vi "Multiprocessing_VI_Latest.vi"() -> ()   [LabVIEW 2022 SP3]
uses:
  <vilib>/Analysis/baseanly.llb/Mean (DBL).vi
  <vilib>/DAQmx/read.llb/DAQmx Read (Analog 1D Wfm NChan NSamp).vi
  STOP_GLOBAL.vi
  <vilib>/DAQmx/configure/timing.llb/DAQmx Timing (Sample Clock).vi
  <vilib>/addons/control/pid/pid.llb/PID Gain Schedule (DBL).vi
  <vilib>/DAQmx/miscellaneous.llb/DAQmx Fill In Error Info.vi
  <resource>/objmgr/daqmx.rc
  <vilib>/addons/control/pid/NI_PID_pid.lvlib
  <vilib>/Analysis/NI_AALBase.lvlib
panel:
  in  "Manual Angle Control":dbl
  out "Voltage":dbl
  out "Waveform Graph":dbl[](graph)
  out "Voltage Command Output":dbl[](graph)
  out "VoltageSent":dbl
  out "Angle Command":dynamicdata(graph)
  in  "Ignition":bool
  in  "Stepper Voltage":ext format="%_3g"
  out "Chamber Pressure LocalVar":dynamicdata(graph)
  out "PID gains out":T1={"proportional gain (Kc)"=1.0, "integral time (Ti, min)"=0.01, "derivative time (Td, min)"=0.0} {"derivative time (Td, min)" format="%.3f"; "integral time (Ti, min)" format="%.5f"; "proportional gain (Kc)" format="%.3f"}
  out "Process Variable vs Setpoint":dynamicdata(graph)
  out "Output":dbl(slide)=30.8641975308642 scale=0.0..5.067 scale format="%.1f"
  in  "Automatic":bool=TRUE
  out "Servo/Step Voltage":dbl[](array[numeric])
  in  "SP":dbl
  in  "MV":dbl(slide)=30.8641975308642 scale=0.0..5.067 scale format="%.1f"
  in  "Stop All":bool
  out "x*y 2":dbl
  out "AI7":dynamicdata(graph)
  out "Time":dbl
  out "Inlet Thermocouple":cluster{dbl[], dbl[]}(graph)
  out "Inlet Thermocouple":dynamicdata(graph)
  out "Flow Meter Thermocouple":dynamicdata(graph)
  out "Supply P. Thermocouple":cluster{dbl[], dbl[]}(graph)
  out "Flow Meter Thermocouple":cluster{dbl[], dbl[]}(graph)
  out "Supply P. Thermocouple":dynamicdata(graph)
  out "Thrust 3":cluster{dbl[], dbl[]}(graph)
  out "Thrust 2":cluster{dbl[], dbl[]}(graph)
  out "Rocket Thrust":cluster{dbl[], dbl[]}(graph)
  out "LC3":dynamicdata(graph)
  out "LC2":dynamicdata(graph)
  out "Rocket Thrust LC1":dynamicdata(graph)
  out "Waiting \nfor Start":bool=TRUE
  in  "Start VI":bool
  out "SampClk.Rate":dbl
  in  "Sample Number":i32=100
  in  "Channel Control":bool[](array[boolean])
  in  "Rate":dbl=1000.0 format="%0.2f"
  out "AI7":cluster{dbl[], dbl[]}(graph)
  out "Vol Flow L/min":dynamicdata(graph)
  out "Process Variable vs Setpoint":cluster{dbl[], dbl[]}[](graph)
  in  "Filename":path=path "C:/1. Rocket Research Project/CollectedData/Plots/TestingData.lvm"
  in  "PID gain schedule":T2(array[cluster])=[{"PID gains"={"proportional gain (Kc)"=1.0, "integral time (Ti, min)"=0.01, "derivative time (Td, min)"=0.0}, "max value"=100.0}] {"max value" format="%.2f"; "PID gains"."derivative time (Td, min)" format="%.3f"; "PID gains"."integral time (Ti, min)" format="%.3f"; "PID gains"."proportional gain (Kc)" format="%.3f"}
  in  "Collect?":bool=TRUE caption="Enable"
  out "Vol Flow":cluster{dbl[], dbl[]}(graph)
  out "Chamber Pressure":cluster{dbl[], dbl[]}(graph)
  out "Inlet Pressure":cluster{dbl[], dbl[]}(graph)
  out "Line Pressure":cluster{dbl[], dbl[]}(graph)
  out "Supply Pressure":cluster{dbl[], dbl[]}(graph)
  out "Supply Pressure":dynamicdata(graph)
  out "Inlet Pressure":dynamicdata(graph)
  out "Line Pressure":dynamicdata(graph)
  out "Chamber Pressure PSI":dynamicdata(graph)
  out "Output Clock Rate":dbl
  out "x*y":i32
  out "error out":errorcluster
  out "Iterations":i32
  out "Angle Sensor":dynamicdata(graph)
  out "P.T. 5":dynamicdata(graph)
  # "Pressure Channels"
  # "Temperature Channels"
  # "Thrust Channels"
  # "DAQ Configuration"
  # "AI 0 - Supply Pressure"
  # "AI 1 - Flow Meter Pressure"
  # "AI 2 - Inlet Pressure"
  # "AI 3 - Chamber Pressure"
  # "AI 4 - Differential Pressure"
  # "AI 5 - Volumetric Flow"
  # "AI 6"
  # "AI 7"
  # "Load Cell 1 Right"
  # "Load Cell 2 Left"
  # "Thrust Channel 3"
  # "TC1 - Supply P. Thermocouple"
  # "TC2 - Flow Meter Thermocouple"
  # "TC3 - Inlet Thermocouple"
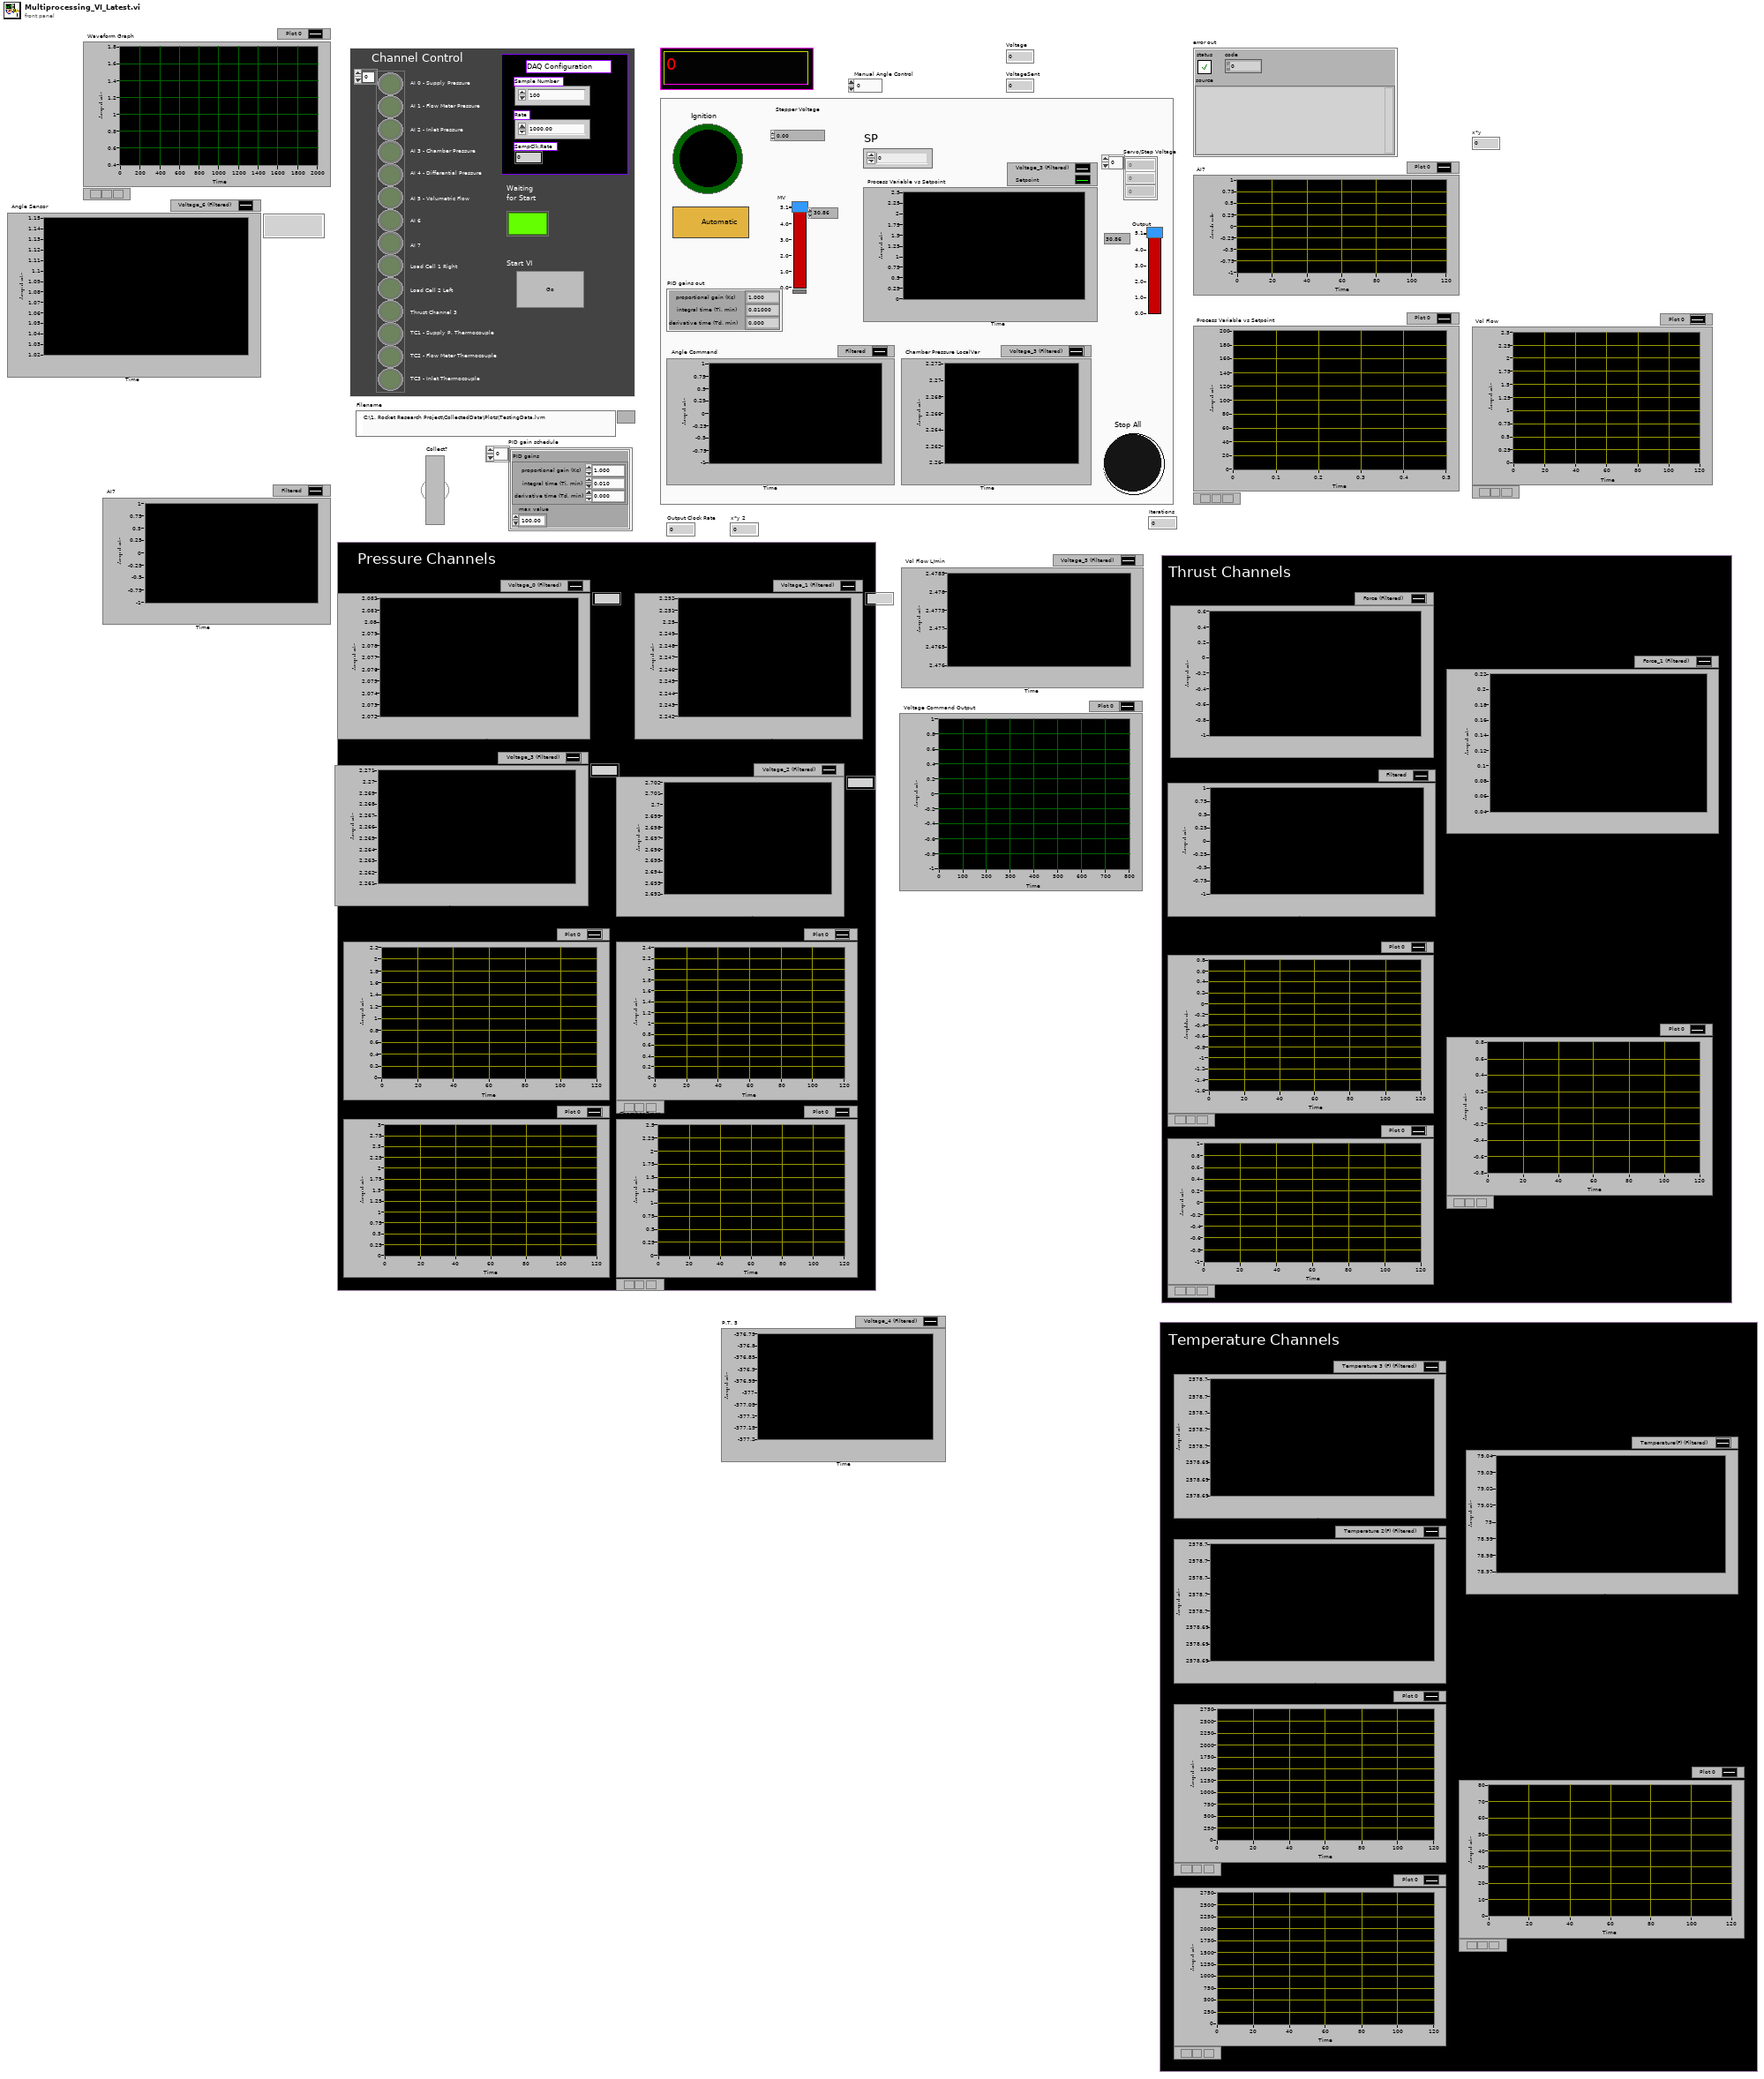
[diagram p1: front panel]
types:
  T1 = cluster{"proportional gain (Kc)":dbl, "integral time (Ti, min)":dbl, "derivative time (Td, min)":dbl}
  T2 = cluster{"PID gains":cluster{"proportional gain (Kc)":dbl, "integral time (Ti, min)":dbl, "derivative time (Td, min)":dbl}, "max value":dbl}[]
  T3 = cluster{"PID gains":cluster{"Kc":dbl, "Ti":dbl, "Td":dbl}, "max value":dbl}[]
  T4 = cluster{"Modulus":dbl, "Number of\nComplete Cycles":dbl}
  T5 = cluster{"Dynamic Data":dynamicdata, "Dynamic Data":dynamicdata, "Dynamic Data":dynamicdata, "Dynamic Data":dynamicdata, "Dynamic Data":dynamicdata, "Dynamic Data":dynamicdata, "Dynamic Data":dynamicdata, "Dynamic Data":dynamicdata, "Dynamic Data":dynamicdata, "Dynamic Data":dynamicdata, "Dynamic Data":dynamicdata, "Dynamic Data":dynamicdata, "Dynamic Data":dynamicdata, "Dynamic Data":dynamicdata}
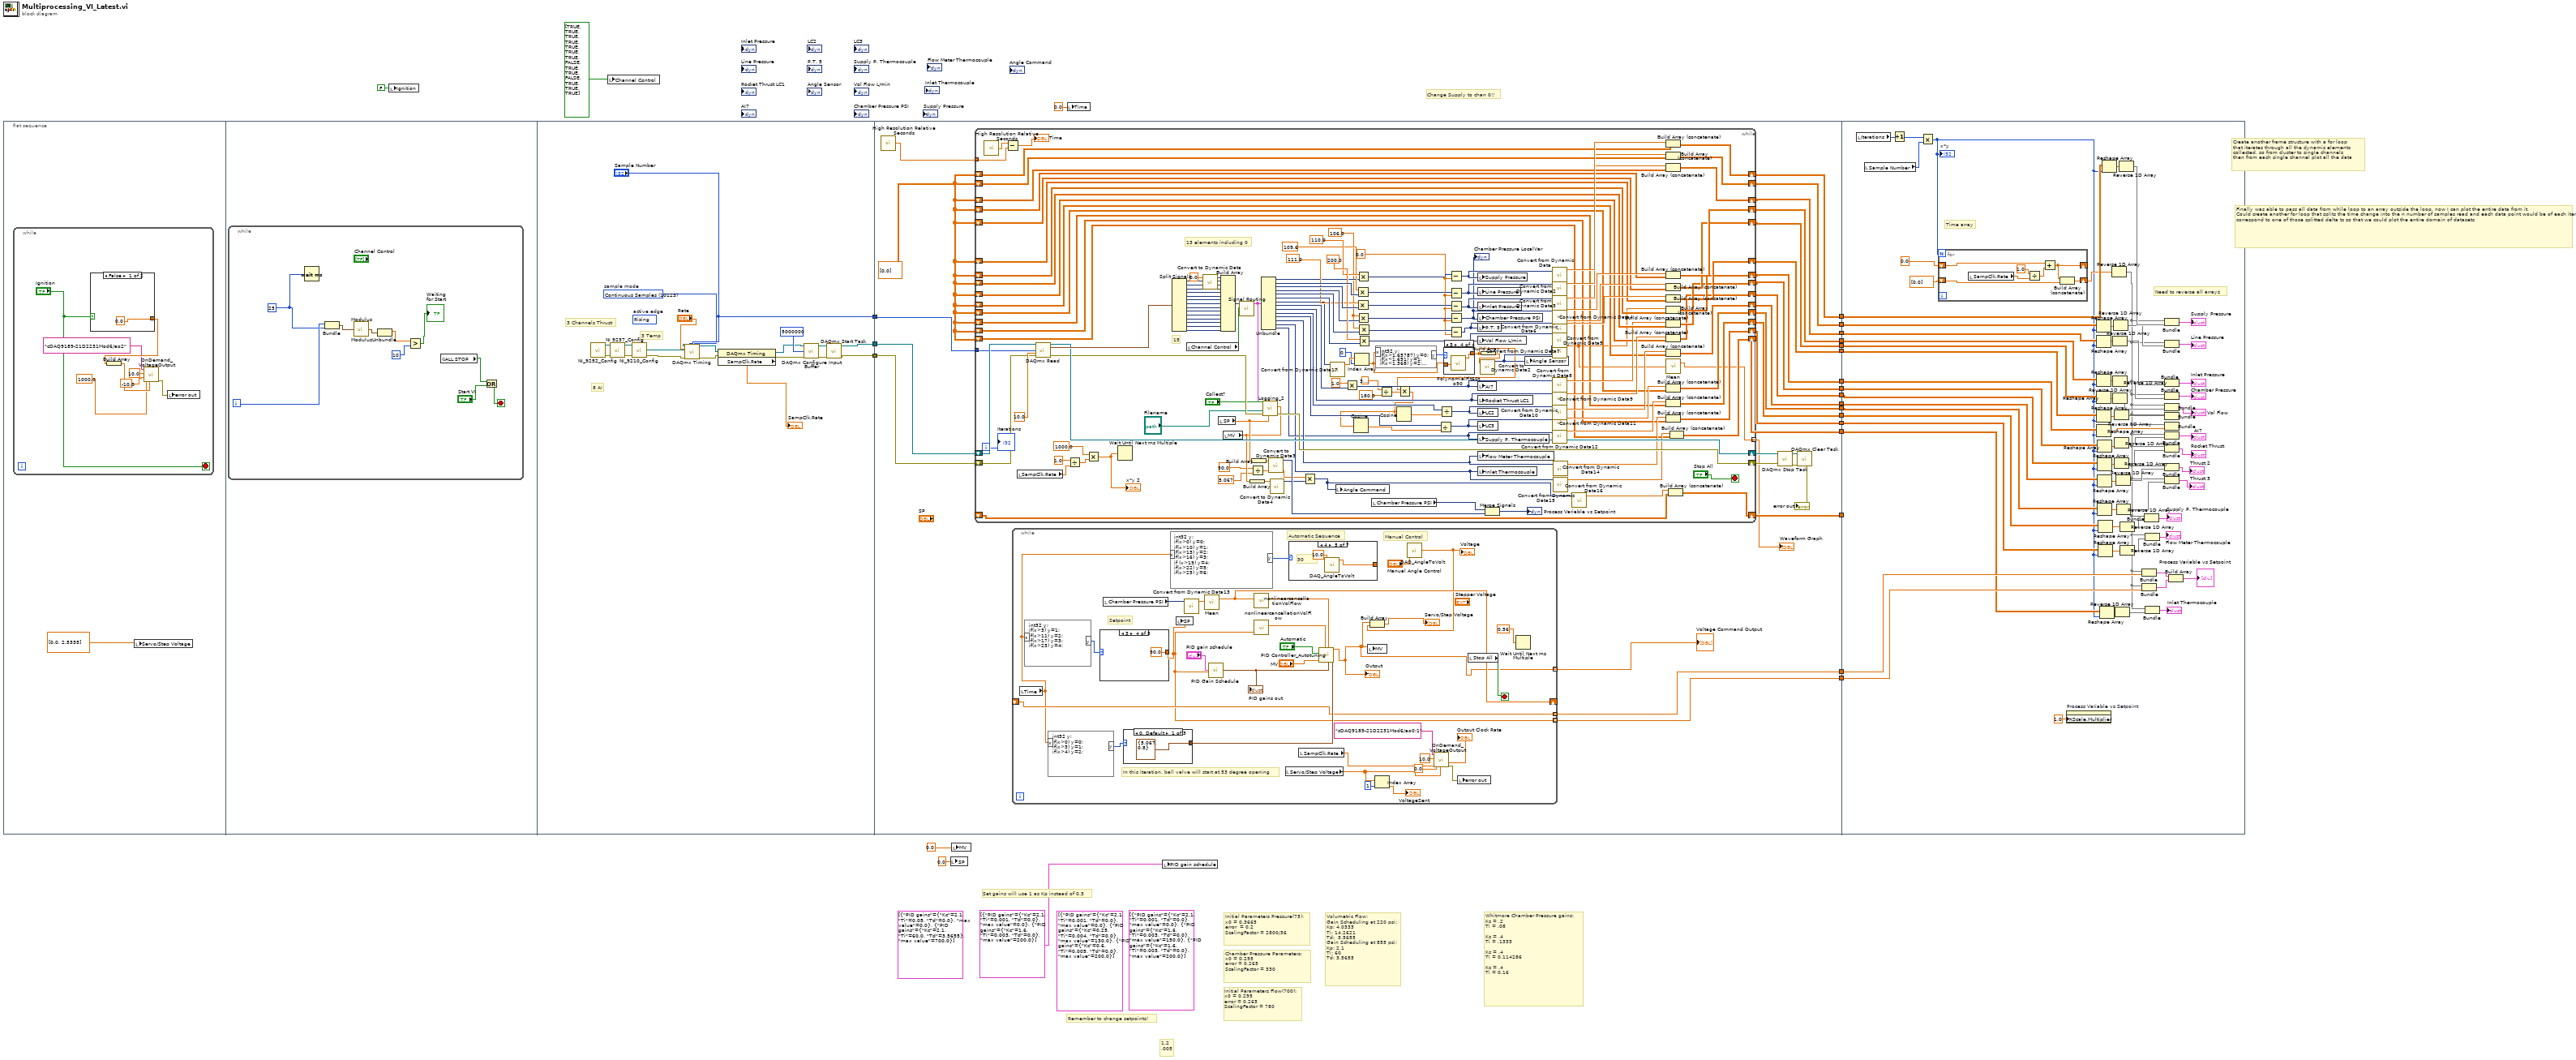
[diagram p0: block diagram]
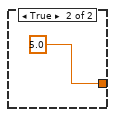
[diagram p2: hidden frame]
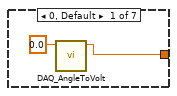
[diagram p3: hidden frame]
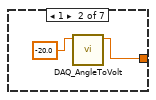
[diagram p4: hidden frame]
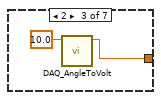
[diagram p5: hidden frame]
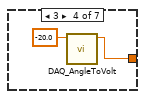
[diagram p6: hidden frame]
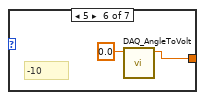
[diagram p7: hidden frame]
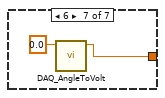
[diagram p8: hidden frame]
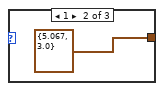
[diagram p9: hidden frame]
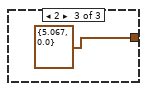
[diagram p10: hidden frame]
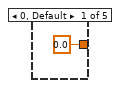
[diagram p11: hidden frame]
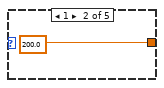
[diagram p12: hidden frame]
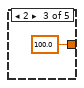
[diagram p13: hidden frame]
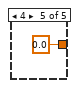
[diagram p14: hidden frame]
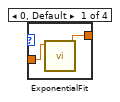
[diagram p15: hidden frame]
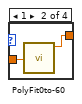
[diagram p16: hidden frame]
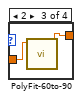
[diagram p17: hidden frame]
diagram:
  (unwired) T3 [{"PID gains"={"Kc"=2.1, "Ti"=0.001, "Td"=0.0}, "max value"=0.0}, {"PID gains"={"Kc"=1.6, "Ti"=0.003, "Td"=0.0}, "max value"=150.0}, {"PID gains"={"Kc"=1.6, "Ti"=0.003, "Td"=0.0}, "max value"=200.0}]
  (unwired) T3 [{"PID gains"={"Kc"=2.1, "Ti"=0.001, "Td"=0.0}, "max value"=0.0}, {"PID gains"={"Kc"=0.25, "Ti"=0.004, "Td"=0.0}, "max value"=130.0}, {"PID gains"={"Kc"=0.6, "Ti"=0.005, "Td"=0.0}, "max value"=200.0}]
  (unwired) T3 [{"PID gains"={"Kc"=2.1, "Ti"=0.05, "Td"=0.0}, "max value"=0.0}, {"PID gains"={"Kc"=2.1, "Ti"=60.0, "Td"=3.5655}, "max value"=700.0}]
  # "1.2\n.005"
  # "Set gains will use 1 as Kp instead of 0.3"
  # "Remember to change setpoints!"
  # "Whitmore Chamber Pressure gains:\nKc = .2\nTi = .08\n\nKc = .4\nTi = .1333\n\nKc = .4\nTi = 0.114286\n\nKc = .4\nTi = 0.16"
  # "Chamber Pressure Parameters:\nx0 = 0.295\nerror = 0.265\nScalingFactor = 330"
  # "Volumetric Flow:\nGain Scheduling at 220 psi:\nKp: 4.0333\nTi: 14.2621\nTd:  3.5655\nGain Scheduling at 855 psi:\nKp: 2.1\nTi: 60\nTd: 3.5655"
  # "Initial Parameters Flow(700):\nx0 = 0.295\nerror = 0.265\nScalingFactor = 780"
  # "Initial Parameters Pressure(75):\nx0 = 0.3665\nerror  = 0.2\nScalingFactor = 2800/36"
  # "Change Supply to chan 0!!"
  # "Finally was able to pass all data from while loop to an array outside the loop, now I can plot the entire data from it, \nCould create another for loop that splits the time change into the n number of samples read and each data point would be of each iteration would correspond to one of those splitted delta ts so that we could plot the entire domain of datasets"
  # "Create another frame structure with a for loop\nthat iterates through all the dynamic elements\ncollected, so from cluster to single channels\nthen from each single channel plot all the data"
  n1 = flat-sequence {
    tunnel: [w59] -> w25
    tunnel: [w48] -> w24
    tunnel: ["Sample Number"] -> w4
    tunnel: w25 -> [w95]
    tunnel: w24 -> [w94]
    tunnel: [w87] -> w23
    tunnel: [w86] -> w21
    tunnel: [w85] -> w20
    tunnel: [w84] -> w19
    tunnel: [w83] -> w18
    tunnel: [w82] -> w17
    tunnel: [w81] -> w16
    tunnel: [w80] -> w15
    tunnel: [w79] -> w14
    tunnel: [w78] -> w13
    tunnel: [w77] -> w12
    tunnel: [w76] -> w11
    tunnel: [w75] -> w9
    tunnel: [w74] -> w8
    tunnel: [w72] -> w6
    tunnel: [w71] -> w5
    tunnel: w4 -> [w70]
    tunnel: [w69] -> w2
    tunnel: w23 -> [w363]
    tunnel: w21 -> [w362]
    tunnel: w20 -> [w361]
    tunnel: w19 -> [w360]
    tunnel: w18 -> [w359]
    tunnel: w17 -> [w358]
    tunnel: w16 -> [w357]
    tunnel: w15 -> [w355]
    tunnel: w14 -> [w354]
    tunnel: w13 -> [w353]
    tunnel: w12 -> [w352]
    tunnel: w11 -> [w351]
    tunnel: w9 -> [w346]
    tunnel: w8 -> [w345]
    tunnel: w6 -> [w320]
    tunnel: w5 -> [w319]
    tunnel: w2 -> [_]
    frame #0 {
      n2 = while {
        stop <- "Ignition" stop-if-true
        n3 = case shown="False" "Ignition" {
          tunnel: [0.0 ("element") 5.0 ("element")] -> w34
          frame False {
          }
          frame True {
          }
        }
        n4 = Build Array(w34) -> (w35:dbl[])
        n5 = call "OnDemand_VoltageOutput.vi"("Channel Array"=w35, "SampClk.Rate 2"=1000.0, "minimum voltage"=-10.0, "maximum voltage"=10.0, "physical channels"="cDAQ9189-21D2231Mod6/ao2") -> ("error out"=w33:errorcluster)  [unwired: 4 in, 2 out]
        n6 = local write "error out"(w33) -> ()
      }
      n7 = local write "Servo/Step Voltage"(dbl[] [0.0, 2.5335] ("Servo/Step Voltage")) -> ()
    }
    frame #1 {
      n8 = while {
        i -> [w47]
        stop <- w39 stop-if-true
        w38 = u32 25 ("milliseconds to wait")
        n9 = Wait (ms)(milliseconds to wait=w38) -> ()  [unwired: 1 out]
        n10 = Bundle(w47, "milliseconds to wait"=w38) -> (w46:cluster{i32, "milliseconds to wait":u32})  [unwired: 1 in]
        n11 = call "Modulus.vi"("Input"=w46) -> ("Output"=w45:T4)
        n12 = call "Modulus.vi"() -> ()  [unwired: 1 in, 1 out]
        n13 = Unbundle(w45) -> ("Modulus"=w44:dbl)  [unwired: 1 out]
        n14 = Greater?(x=w44, y=u32 10 ("milliseconds to wait")) -> (0:→"Waiting \nfor Start":bool)
        n15 = global read "STOP_GLOBAL.vi" "ALL STOP"() -> (w41:bool)
        n16 = Or(x=w41, y="Start VI") -> (x .or. y?=w39:bool)
      }
    }
    frame #2 {
      w50 = 10123 items=["Finite Samples"=10178, "Continuous Samples"=10123, "Hardware Timed Single Point"=12522]  # sample mode
      (unwired) 10280 items=["Rising"=10280, "Falling"=10171]  # active edge
      # "3 Temp"
      # "8 AI"
      # "3 Channels Thrust"
      n17 = call "NI_9252_Config.vi"() -> ("error out"=w57:errorcluster, "task out"=w58:refnum<k21>)  [unwired: 10 in]
      n18 = call "NI 9237_Config.vi"("error in"=w57, "task in"=w58) -> ("error out"=w66:errorcluster, "task out"=w65:refnum<k21>)  [unwired: 8 in]
      n19 = call "NI_9210_Config.vi"("error in"=w66, "task in"=w65) -> ("error out"=w53:errorcluster, "task out"=w55:refnum<k21>)  [unwired: 8 in]
      n20 = call-poly <vilib>:"DAQmx Timing.vi"("task/channels in"=w55, "sample mode"=w50, "samples per channel"="Sample Number", "rate"="Rate", "error in"=w53) -> ("task out"=w51:refnum<k21>, "error out"=w52:errorcluster)  [unwired: 9 in]
      n21 = property class="DAQmx Timing"(reference=w51, error in=w52) -> (reference out=w49:refnum<k21>, error out=w62:errorcluster, "SampClk.Rate"=→"SampClk.Rate":dbl)
      n22 = call <vilib>:"DAQmx Configure Input Buffer.vi"("task/channels in"=w49, "buffer size (in samples per channel)"=u32 5000000, "error in"=w62) -> ("task out"=w64:refnum<k21>, "error out"=w63:errorcluster)  [unwired: 11 in]
      n23 = call <vilib>:"DAQmx Start Task.vi"("task/channels in"=w64, "error in"=w63) -> ("task out"=w59:refnum<k21>, "error out"=w48:errorcluster)  [unwired: 12 in]
    }
    frame #3 {
      w73 = dbl[][] [[0.0]]
      n24 = call <vilib>:"High Resolution Relative Seconds.vi"() -> ("relative seconds"=w93:dbl)
      n25 = while {
        shift-right: [w289] -> w89
        shift-left: w95 -> [w291]
        shift-right: [w267] -> w88
        shift-left: w94 -> [w290]
        shift-right: [w178] -> w87
        shift-left: w73 -> [w227]
        tunnel: w93 -> [w264]
        shift-right: [w258] -> w86
        shift-left: w73 -> [w259]
        shift-right: [w254] -> w85
        shift-left: w73 -> [w255]
        shift-right: [w252] -> w84
        shift-left: w73 -> [w253]
        shift-right: [w250] -> w83
        shift-left: w73 -> [w249]
        shift-right: [w247] -> w82
        shift-left: w73 -> [w245]
        shift-right: [w246] -> w81
        shift-left: w73 -> [w244]
        shift-right: [w243] -> w80
        shift-left: w73 -> [w242]
        shift-right: [w237] -> w79
        shift-left: w73 -> [w236]
        shift-right: [w235] -> w78
        shift-left: w73 -> [w234]
        shift-right: [w232] -> w77
        shift-left: w73 -> [w231]
        shift-right: [w229] -> w76
        shift-left: w73 -> [w228]
        shift-right: [w206] -> w72
        shift-left: w73 -> [w205]
        shift-right: [w202] -> w71
        shift-left: w73 -> [w203]
        tunnel: w70 -> [w199]
        shift-right: [w173] -> w69
        shift-left: _ -> [w174]
        tunnel: [w167] -> w67 mode=indexing
        i -> [w266]
        stop <- "Stop All" stop-if-true
        w169 = 106.0 ("x")
        w191 = 0.0 ("y")
        # "13 elements including 0"
        # "15"
        n26 = call <vilib>:"High Resolution Relative Seconds.vi"() -> ("relative seconds"=w265:dbl)
        n27 = Subtract(x=w265, y=w264) -> (x-y=→"Time":dbl)
        n28 = local read "SampClk.Rate"() -> (w224:dbl)
        n29 = call-poly <vilib>:"DAQmx Read.vi"("task/channels in"=w291, "number of samples per channel"=w199, "timeout"=10.0, "error in"=w290) -> ("task out"=w289:refnum<k21>, "data"=w292:waveform(dbl)[], "error out"=w269:errorcluster)  [unwired: 9 in]
        n30 = Divide(x=1.0, y=w224) -> (x/y=w223:dbl)
        n31 = Multiply(x=1000.0, y=w223) -> (x*y=w221:dbl)
        "x*y 2" <- w221
        n32 = Wait Until Next ms Multiple(millisecond multiple=w221) -> ()  [unwired: 1 out]
        n33 = Split Signals(w292) -> (w283:dynamicdata, w288:dynamicdata, w287:dynamicdata, w286:dynamicdata, w285:dynamicdata, w284:dynamicdata, w282:dynamicdata, w281:dynamicdata, w280:dynamicdata, w279:dynamicdata, w278:dynamicdata, w275:dynamicdata, w209:dynamicdata, w208:dynamicdata)  [unwired: 14 in]
        n34 = local read "Channel Control"() -> (w274:bool[])
        n35 = call "Convert to Dynamic Data"("Double"=0.0) -> ("Dynamic Data Type"=w276:dynamicdata)  [unwired: 3 in]
        n36 = local read "SP"() -> (w189:dbl)
        n37 = Build Array(w276, w283, w288, w287, w286, w285, w284, w282, w281, w280, w279, w278, w275, w209, w208) -> (w273:dynamicdata[])
        n38 = local read "MV"() -> (w184:dbl)
        n39 = call "Signal Routing.vi"("Boolean Array"=w274, "Data In"=w273) -> ("Output"=w198:T5)  [unwired: 9 in]
        n40 = Build Array(w184) -> (w183:dbl[])
        n41 = Divide(x=90.0, y=5.067) -> (x/y=w172:dbl)
        n42 = Build Array(w189) -> (w188:dbl[])
        n43 = Unbundle(w198) -> ("Dynamic Data"=w177:dynamicdata, "Dynamic Data"=w272:dynamicdata, "Dynamic Data"=w271:dynamicdata, "Dynamic Data"=w190:dynamicdata, "Dynamic Data"=w270:dynamicdata, "Dynamic Data"=w201:dynamicdata, "Dynamic Data"=w155:dynamicdata, "Dynamic Data"=w220:dynamicdata, "Dynamic Data"=w241:dynamicdata, "Dynamic Data"=w160:dynamicdata, "Dynamic Data"=w157:dynamicdata, "Dynamic Data"=w197:dynamicdata, "Dynamic Data"=w195:dynamicdata, "Dynamic Data"=w196:dynamicdata)
        n44 = call "Logging_2.vi"("Voltage Command"=w184, "Setpoint"=w189, "error in"=w269, "Filename"="Filename", "Enable"="Collect?", "output cluster"=w198) -> ("error out"=w267:errorcluster)  [unwired: 5 in]
        n45 = call "Convert to Dynamic Data3"("Array"=w188) -> ("Dynamic Data Type"=w187:dynamicdata)  [unwired: 3 in]
        n46 = call "Convert to Dynamic Data4"("Array"=w183) -> ("Dynamic Data Type"=w182:dynamicdata)  [unwired: 3 in]
        n47 = Multiply(x=w172, y=w182) -> (x*y=w176:dynamicdata)
        n48 = call "Convert from Dynamic Data17"("Dynamic Data Type"=w155) -> ("Array"=w165:dbl[])  [unwired: 3 in]
        n49 = local write "Angle Command"(w176) -> ()
        n50 = Multiply(x=1.0, y=w220) -> (x*y=w218:dynamicdata)
        n51 = Index Array(array=w165, index=0) -> (element=w162:dbl)
        n52 = Multiply(x=109.6, y=w272) -> (x*y=w216:dynamicdata)
        n53 = Multiply(x=111.0, y=w271) -> (x*y=w217:dynamicdata)
        n54 = Multiply(x=110.0, y=w177) -> (x*y=w215:dynamicdata)
        n55 = Multiply(x=w169, y=w190) -> (x*y=w211:dynamicdata)
        n56 = Multiply(x=w169, y=w270) -> (x*y=w193:dynamicdata)
        n57 = Multiply(x=200.0, y=w201) -> (x*y=w194:dynamicdata)
        n58 = local read "Chamber Pressure PSI"() -> (w185:dynamicdata)
        n59 = formula code="int32 y;\nif(x>1.65787) y=0;\nif(x<1.651) y=1;\nif(x<1.368) y=2;\nif(x>1.935) y=3;"("x"=w162) -> ("y"=w166:i32)
        n60 = Divide(x=3.141592653589793, y=180.0 ("x")) -> (x/y=w151:dbl)
        n61 = case shown="3" w166 {
          tunnel: w162 -> [w295 w297 w299 w301]
          tunnel: [w294 w296 w298 w300] -> w150
          frame 0, Default {
            n62 = call "ExponentialFit.vi"("voltage"=w295) -> ("angle"=w294:dbl)  [unwired: 10 in]
          }
          frame 1 {
            n63 = call "PolyFit0to-60.vi"("input variable"=w297) -> ("output variable"=w296:dbl)  [unwired: 10 in]
          }
          frame 2 {
            n64 = call "PolyFit-60to-90.vi"("Voltage"=w299) -> ("Angle"=w298:dbl)  [unwired: 10 in]
          }
          frame 3 {
            n65 = call "PolynomialFit60to90.vi"("voltage"=w301) -> ("Angle"=w300:dbl)  [unwired: 10 in]
          }
        }
        n66 = Multiply(x=w150, y=w151) -> (x*y=w149:dbl)
        n67 = Cosine(x=w149) -> (cos(x)=w158:dbl)
        n68 = Cosine(x=w149) -> (cos(x)=w161:dbl)
        n69 = Divide(x=w157, y=w158) -> (x/y=w156:dynamicdata)
        n70 = Divide(x=w160, y=w161) -> (x/y=w159:dynamicdata)
        n71 = Subtract(x=w215, y=w191) -> (x-y=w214:dynamicdata)
        n72 = Subtract(x=w216, y=w191) -> (x-y=w213:dynamicdata)
        n73 = Subtract(x=w217, y=w191) -> (x-y=w212:dynamicdata)
        n74 = Subtract(x=w211, y=w191) -> (x-y=w210:dynamicdata)
        "Chamber Pressure LocalVar" <- w210
        n75 = Subtract(x=w193, y=w191) -> (x-y=w192:dynamicdata)
        n76 = local write "Supply Pressure"(w214) -> ()
        n77 = local write "Line Pressure"(w213) -> ()
        n78 = local write "Inlet Pressure"(w212) -> ()
        n79 = local write "Chamber Pressure PSI"(w210) -> ()
        n80 = local write "P.T. 5"(w192) -> ()
        n81 = local write "Vol Flow L/min"(w194) -> ()
        n82 = local write "AI7"(w218) -> ()
        n83 = local write "Rocket Thrust LC1"(w241) -> ()
        n84 = local write "LC2"(w159) -> ()
        n85 = local write "LC3"(w156) -> ()
        n86 = local write "Supply P. Thermocouple"(w196) -> ()
        n87 = local write "Flow Meter Thermocouple"(w197) -> ()
        n88 = local write "Inlet Thermocouple"(w195) -> ()
        n89 = Build Array(w150) -> (w163:dbl[])
        n90 = call "Convert to Dynamic Data2"("Array"=w163) -> ("Dynamic Data Type"=w154:dynamicdata)  [unwired: 3 in]
        n91 = Merge Signals(w185, w187) -> (→"Process Variable vs Setpoint":dynamicdata)
        n92 = local write "Angle Sensor"(w154) -> ()
        n93 = call "Convert from Dynamic Data"("Dynamic Data Type"=w214) -> ("Array"=w263:dbl[])  [unwired: 3 in]
        n94 = call "Convert from Dynamic Data2"("Dynamic Data Type"=w213) -> ("Array"=w260:dbl[])  [unwired: 3 in]
        n95 = call "Convert from Dynamic Data3"("Dynamic Data Type"=w212) -> ("Array"=w257:dbl[])  [unwired: 3 in]
        n96 = call "Convert from Dynamic Data4"("Dynamic Data Type"=w210) -> ("Array"=w256:dbl[])  [unwired: 3 in]
        n97 = call "Convert from Dynamic Data6"("Dynamic Data Type"=w192) -> ("Array"=w248:dbl[])  [unwired: 3 in]
        n98 = call "Convert from Dynamic Data5"("Dynamic Data Type"=w194) -> ("Array"=w251:dbl[])  [unwired: 3 in]
        n99 = call "Convert from Dynamic Data7"("Dynamic Data Type"=w154) -> ("Array"=w168:dbl[])  [unwired: 3 in]
        n100 = call "Convert from Dynamic Data8"("Dynamic Data Type"=w218) -> ("Array"=w240:dbl[])  [unwired: 3 in]
        n101 = call "Convert from Dynamic Data9"("Dynamic Data Type"=w241) -> ("Array"=w239:dbl[])  [unwired: 3 in]
        n102 = call "Convert from Dynamic Data10"("Dynamic Data Type"=w159) -> ("Array"=w238:dbl[])  [unwired: 3 in]
        n103 = call "Convert from Dynamic Data11"("Dynamic Data Type"=w156) -> ("Array"=w233:dbl[])  [unwired: 3 in]
        n104 = call "Convert from Dynamic Data12"("Dynamic Data Type"=w196) -> ("Array"=w230:dbl[])  [unwired: 3 in]
        n105 = call "Convert from Dynamic Data14"("Dynamic Data Type"=w197) -> ("Array"=w207:dbl[])  [unwired: 3 in]
        n106 = call "Convert from Dynamic Data15"("Dynamic Data Type"=w195) -> ("Array"=w204:dbl[])  [unwired: 3 in]
        n107 = call "Convert from Dynamic Data16"("Dynamic Data Type"=w176) -> ("Array"=w175:dbl[])  [unwired: 3 in]
        n108 = Build Array (concatenate)(w263, w227) -> (w178:dbl[][])
        n109 = Build Array (concatenate)(w260, w259) -> (w258:dbl[][])
        n110 = Build Array (concatenate)(w257, w255) -> (w254:dbl[][])
        n111 = Build Array (concatenate)(w256, w253) -> (w252:dbl[][])
        n112 = Build Array (concatenate)(w251, w249) -> (w250:dbl[][])
        n113 = Build Array (concatenate)(w248, w245) -> (w247:dbl[][])
        n114 = Build Array (concatenate)(w168, w244) -> (w246:dbl[][])
        n115 = Build Array (concatenate)(w240, w242) -> (w243:dbl[][])
        n116 = Build Array (concatenate)(w239, w236) -> (w237:dbl[][])
        n117 = Build Array (concatenate)(w238, w234) -> (w235:dbl[][])
        n118 = Build Array (concatenate)(w233, w231) -> (w232:dbl[][])
        n119 = Build Array (concatenate)(w230, w228) -> (w229:dbl[][])
        n120 = call-poly <vilib>:"Mean.vi"("X"=w168) -> ("mean"=w167:dbl)  [unwired: 1 out]
        n121 = Build Array (concatenate)(w207, w205) -> (w206:dbl[][])
        n122 = Build Array (concatenate)(w175, w174) -> (w173:dbl[][])
        n123 = Build Array (concatenate)(w204, w203) -> (w202:dbl[][])
        "Iterations" <- w266
      }
      "Waveform Graph" <- w67
      n124 = while {
        shift-right: [w118] -> _
        shift-left: _ -> [w114]
        tunnel: [w114] -> w75 mode=indexing
        tunnel: [w106] -> w74 mode=indexing
        tunnel: [w98] -> w68 mode=indexing
        stop <- w121 stop-if-true
        # "Manual Control"
        # "Automatic Sequence"
        # "In this iteration, ball valve will start at 53 degree opening"
        # "Setpoint"
        n125 = local read "Time"() -> (w103:dbl)
        n126 = formula code="int32 y;\nif(x>3) y=1;\nif(x>11) y=2;\nif(x>17) y=3;\nif(x>23) y=4;"("x"=w103) -> ("y"=w117:i32)
        n127 = formula code="int32 y;\nif(x>0) y=0;\nif(x>3) y=1;\nif(x>4) y=2;"("x"=w103) -> ("y"=w116:i32)
        n128 = case shown="3" w117 {
          tunnel: [0.0 ("SP") 200.0 ("SP") 100.0 ("SP") 90.0 ("SP") 0.0 ("SP")] -> w106
          frame 0, Default {
          }
          frame 1 {
          }
          frame 2 {
          }
          frame 3 {
          }
          frame 4 {
          }
        }
        n129 = local read "Chamber Pressure PSI"() -> (w105:dynamicdata)
        n130 = case shown="0, Default" w116 {
          tunnel: [cluster{"output high":dbl, "output low":dbl} {"output high"=5.067, "output low"=0.8} ("output range") cluster{"output high":dbl, "output low":dbl} {"output high"=5.067, "output low"=3.0} ("output range") cluster{"output high":dbl, "output low":dbl} {"output high"=5.067, "output low"=0.0} ("output range")] -> w115
          frame 0, Default {
          }
          frame 1 {
          }
          frame 2 {
          }
        }
        n131 = formula code="int32 y;\nif(x>0) y=0;\nif(x>10) y=1;\nif(x>13) y=2;\nif(x>16) y=3;\nif (x>19) y=4;\nif(x>22) y=5;\nif(x>25) y=6;"("x"=w103) -> ("y"=w102:i32)
        n132 = local write "SP"(w106) -> ()
        n133 = call "Convert from Dynamic Data13"("Dynamic Data Type"=w105) -> ("Array"=w119:dbl[])  [unwired: 3 in]
        n134 = call-poly <vilib>:"Mean.vi"("X"=w119) -> ("mean"=w118:dbl)  [unwired: 1 out]
        n135 = call-poly <vilib>:"PID Gain Schedule.vi"("PID gain schedule"="PID gain schedule", "gain scheduling value"=w106) -> ("PID gains out"=w125:T1)  [unwired: 2 in, 1 out]
        "PID gains out" <- w125
        n136 = call "nonlinearcancellationVolFlow.vi"("input variable"=w118) -> ("MVT Process Variable"=w120:dbl)  [unwired: 10 in]
        n137 = call "nonlinearcancellationVolFlow.vi"("input variable"=w106) -> ("MVT Process Variable"=w123:dbl)  [unwired: 10 in]
        n138 = local read "Servo/Step Voltage"() -> (w101:dbl[])
        n139 = case shown="4" w102 {
          tunnel: [w128 w129 w131 w134 w135 w138 w139] -> _
          frame 0, Default {
            n140 = call "DAQ_AngleToVolt.vi"("Angle"=0.0) -> ("Voltage"=w128:dbl)  [unwired: 10 in]
          }
          frame 1 {
            n141 = call "DAQ_AngleToVolt.vi"("Angle"=-20.0 ("x")) -> ("Voltage"=w129:dbl)  [unwired: 10 in]
          }
          frame 2 {
            n142 = call "DAQ_AngleToVolt.vi"("Angle"=10.0) -> ("Voltage"=w131:dbl)  [unwired: 10 in]
          }
          frame 3 {
            n143 = call "DAQ_AngleToVolt.vi"("Angle"=-20.0) -> ("Voltage"=w134:dbl)  [unwired: 10 in]
          }
          frame 4 {
            # "30"
            n144 = call "DAQ_AngleToVolt.vi"("Angle"=10.0) -> ("Voltage"=w135:dbl)  [unwired: 10 in]
          }
          frame 5 {
            # "-10"
            n145 = call "DAQ_AngleToVolt.vi"("Angle"=0.0) -> ("Voltage"=w138:dbl)  [unwired: 10 in]
          }
          frame 6 {
            n146 = call "DAQ_AngleToVolt.vi"("Angle"=0.0) -> ("Voltage"=w139:dbl)  [unwired: 10 in]
          }
        }
        n147 = local read "SampClk.Rate"() -> (w112:dbl)
        n148 = call "PID Controller_Autotuning.vi"("output range"=w115, "PID gains in"=w125, "process variable"=w120, "setpoint"=w123, "manipulated variable"="MV", "Automatic"="Automatic") -> ("output"=w98:dbl)  [unwired: 4 in, 1 out]
        "Output" <- w98
        n149 = local write "MV"(w98) -> ()
        n150 = Index Array(array=w101, index=1) -> (element=→"VoltageSent":dbl)
        n151 = call "DAQ_AngleToVolt.vi"("Angle"="Manual Angle Control") -> ("Voltage"=w96:dbl)  [unwired: 10 in]
        "Voltage" <- w96
        n152 = Build Array(w98, w96) -> (→"Servo/Step Voltage":dbl[])
        n153 = call "OnDemand_VoltageOutput.vi"("Channel Array"=w101, "SampClk.Rate 2"=w112, "minimum voltage"=0.0, "maximum voltage"=10.0, "physical channels"="cDAQ9189-21D2231Mod6/ao0:1") -> ("error out"=w111:errorcluster, "SampClk.Rate"=→"Output Clock Rate":dbl)  [unwired: 4 in, 1 out]
        n154 = local write "error out"(w111) -> ()
        n155 = local read "Stop All"() -> (w121:bool)
        n156 = Wait Until Next ms Multiple(millisecond multiple=0.56 ("x")) -> ()  [unwired: 1 out]
      }
      "Voltage Command Output" <- w68
      n157 = call <vilib>:"DAQmx Stop Task.vi"("task/channels in"=w89, "error in"=w88) -> ("task out"=w92:refnum<k21>, "error out"=w91:errorcluster)  [unwired: 12 in]
      n158 = call <vilib>:"DAQmx Clear Task.vi"("task in"=w92, "error in"=w91) -> ("error out"=→"error out":errorcluster)  [unwired: 13 in]
    }
    frame #4 {
      # "Time array"
      # "Need to reverse all arrays"
      n159 = local read "Iterations"() -> (w368:i32)
      n160 = local read "Sample Number"() -> (w304:i32)
      n161 = Increment(x=w368) -> (x+1=w367:i32)
      n162 = Multiply(x=w367, y=w304) -> (x*y=w303:i32)
      "x*y" <- w303
      n163 = for {
        N: w303 -> [_]
        shift-right: [w371] -> _
        shift-left: 0.0 -> [w372]
        shift-right: [w370] -> w341
        shift-left: dbl[] [0.0] -> [w369]
        n164 = local read "SampClk.Rate"() -> (w374:dbl)
        n165 = Divide(x=1.0, y=w374) -> (x/y=w373:dbl)
        n166 = Add(x=w372, y=w373) -> (x+y=w371:dbl)
        n167 = Build Array (concatenate)(w371, w369) -> (w370:dbl[])
      }
      n168 = property on="Process Variable vs Setpoint" class="XYGraph (strict)"("XScale.Multiplier"=1.0 ("X Scale.Offset and Multiplier:Multiplier")) -> ()  [unwired: 2 in, 2 out]
      n169 = Reshape Array(w362, w303) -> (w337:dbl[])
      n170 = Reshape Array(w361, w303) -> (w335:dbl[])
      n171 = Reshape Array(w360, w303) -> (w333:dbl[])
      n172 = Reshape Array(w359, w303) -> (w331:dbl[])
      n173 = Reshape Array(w358, w303) -> (w329:dbl[])
      n174 = Reshape Array(w357, w303) -> (w356:dbl[])
      n175 = Reshape Array(w355, w303) -> (w326:dbl[])
      n176 = Reshape Array(w353, w303) -> (w310:dbl[])
      n177 = Reshape Array(w354, w303) -> (w318:dbl[])
      n178 = Reshape Array(w352, w303) -> (w307:dbl[])
      n179 = Reshape Array(w351, w303) -> (w323:dbl[])
      n180 = Reshape Array(w320, w303) -> (w316:dbl[])
      n181 = Reshape Array(w319, w303) -> (w311:dbl[])
      n182 = Reshape Array(w363, w303) -> (w339:dbl[])
      n183 = Reverse 1D Array(array=w341) -> (reversed array=w302:dbl[])
      n184 = Reverse 1D Array(array=w335) -> (reversed array=w334:dbl[])
      n185 = Reverse 1D Array(array=w333) -> (reversed array=w332:dbl[])
      n186 = Reverse 1D Array(array=w331) -> (reversed array=w330:dbl[])
      n187 = Reverse 1D Array(array=w337) -> (reversed array=w336:dbl[])
      n188 = Reverse 1D Array(array=w329) -> (reversed array=w328:dbl[])
      n189 = Reverse 1D Array(array=w318) -> (reversed array=w317:dbl[])
      n190 = Reverse 1D Array(array=w326) -> (reversed array=w325:dbl[])
      n191 = Reverse 1D Array(array=w311) -> (reversed array=w312:dbl[])
      n192 = Reverse 1D Array(array=w310) -> (reversed array=w309:dbl[])
      n193 = Reverse 1D Array(array=w307) -> (reversed array=w306:dbl[])
      n194 = Reverse 1D Array(array=w339) -> (reversed array=w338:dbl[])
      n195 = Reverse 1D Array(array=w323) -> (reversed array=w322:dbl[])
      n196 = Reverse 1D Array(array=w316) -> (reversed array=w315:dbl[])
      n197 = Bundle(w302, w346) -> (w343:cluster{dbl[], dbl[]})  [unwired: 1 in]
      n198 = Bundle(w302, w345) -> (w344:cluster{dbl[], dbl[]})  [unwired: 1 in]
      n199 = Bundle(w302, w322) -> (→"Supply P. Thermocouple":cluster{dbl[], dbl[]})  [unwired: 1 in]
      n200 = Bundle(w302, w315) -> (→"Flow Meter Thermocouple":cluster{dbl[], dbl[]})  [unwired: 1 in]
      n201 = Bundle(w302, w312) -> (→"Inlet Thermocouple":cluster{dbl[], dbl[]})  [unwired: 1 in]
      n202 = Bundle(w302, w338) -> (→"Supply Pressure":cluster{dbl[], dbl[]})  [unwired: 1 in]
      n203 = Bundle(w302, w336) -> (→"Line Pressure":cluster{dbl[], dbl[]})  [unwired: 1 in]
      n204 = Bundle(w302, w334) -> (→"Inlet Pressure":cluster{dbl[], dbl[]})  [unwired: 1 in]
      n205 = Bundle(w302, w332) -> (→"Chamber Pressure":cluster{dbl[], dbl[]})  [unwired: 1 in]
      n206 = Bundle(w302, w330) -> (→"Vol Flow":cluster{dbl[], dbl[]})  [unwired: 1 in]
      n207 = Bundle(w302, w328) -> ()  [unwired: 1 in, 1 out]
      n208 = Bundle(w302, w356) -> ()  [unwired: 1 in, 1 out]
      n209 = Bundle(w302, w325) -> (→"AI7":cluster{dbl[], dbl[]})  [unwired: 1 in]
      n210 = Bundle(w302, w317) -> (→"Rocket Thrust":cluster{dbl[], dbl[]})  [unwired: 1 in]
      n211 = Bundle(w302, w309) -> (→"Thrust 2":cluster{dbl[], dbl[]})  [unwired: 1 in]
      n212 = Bundle(w302, w306) -> (→"Thrust 3":cluster{dbl[], dbl[]})  [unwired: 1 in]
      n213 = Build Array(w343, w344) -> (→"Process Variable vs Setpoint":cluster{dbl[], dbl[]}[])
    }
  }
  n214 = local write "Ignition"(FALSE ("Ignition")) -> ()
  n215 = local write "Channel Control"(bool[] [TRUE, TRUE, TRUE, TRUE, TRUE, TRUE, TRUE, FALSE, TRUE, TRUE, FALSE, TRUE, TRUE, TRUE] ("Array")) -> ()
  n216 = local write "SP"(0.0 ("SP")) -> ()
  n217 = local write "MV"(0.0 ("MV")) -> ()
  n218 = local write "Time"(0.0 ("Time")) -> ()
  n219 = local write "PID gain schedule"(T3 [{"PID gains"={"Kc"=2.1, "Ti"=0.001, "Td"=0.0}, "max value"=0.0}, {"PID gains"={"Kc"=1.6, "Ti"=0.003, "Td"=0.0}, "max value"=200.0}]) -> ()
